vi "Validate Major Frame.vi"(8 "error in (no error)":errorcluster, 11 "Bus Controller in":refnum<class "Bus Controller.lvclass">) -> (0 "error out":errorcluster, 3 "Bus Controller out":refnum<class "Bus Controller.lvclass">)   [LabVIEW 2016, in "BCI-1553 API.lvlib" / "Bus Controller.lvclass"]
doc: "Checks if the current major frame is default or not. If the class is equivalent to the class default, we initialize a major frame for basic use."
uses:
  Bus Controller.lvclass
  Frames & Messages/Major Frame/Major Frame.lvclass
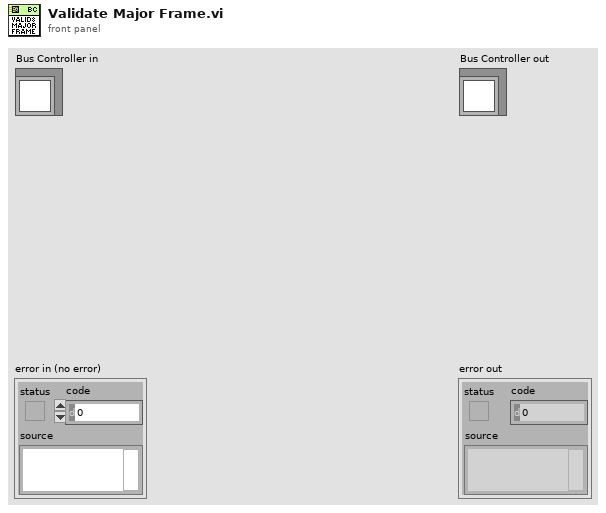
[diagram p1: front panel]
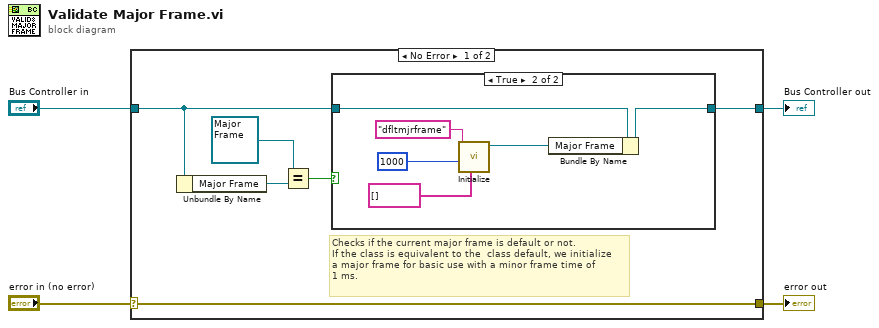
[diagram p0: block diagram]
diagram:
  n1 = case shown="No Error" "error in (no error)" {
    selector: "error in (no error)" -> [w10 w19]
    tunnel: [w10 w19] -> w3
    tunnel: [w6 w18] -> w1
    tunnel: "Bus Controller in" -> [w5 w18]
    frame No Error {
      # "Checks if the current major frame is default or not.\nIf the class is equivalent to the  class default, we initialize\na major frame for basic use with a minor frame time of\n1 ms."
      n2 = Unbundle By Name(w5) -> ("Major Frame"=w9:refnum<class "Major Frame.lvclass">)
      n3 = Equal?(x=refnum<class "Major Frame.lvclass"> refnum ("y"), y=w9) -> (x = y?=w7:bool)
      n4 = case shown="True" w7 {
        tunnel: [w11 w16] -> w6
        tunnel: w5 -> [w11 w17]
        frame False {
        }
        frame True {
          n5 = call "Initialize.vi"("Schedule"=string[] [], "Minor Frame Time (100 us)"=u32 1000, "ID"="dfltmjrframe") -> ("Major Frame out"=w15:refnum<class "Major Frame.lvclass">)  [unwired: 7 in, 1 out]
          n6 = Bundle By Name(cluster=w17, "Major Frame"=w15) -> (w16:refnum<class "Bus Controller.lvclass">)
        }
      }
    }
    frame Error {
    }
  }
  "error out" <- w3
  "Bus Controller out" <- w1
